vi "GetSerialNumber.vi"(8 "error in (no error)":errorcluster) -> (0 "error out":errorcluster, 2 "SerialNumber":string)   [LabVIEW 2014]
uses:
  USBAnalyzerEllisysDll.dll
panel:
  in  "stringOut":string
  in  "sizeOut 2":i32
  out "sizeOut":i32
  in  "return type":i32
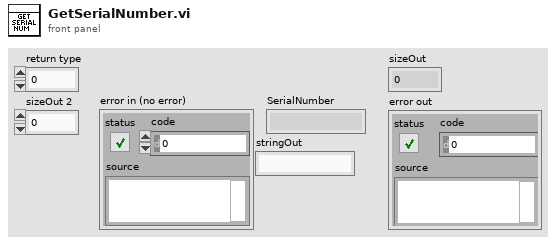
[diagram p1: front panel]
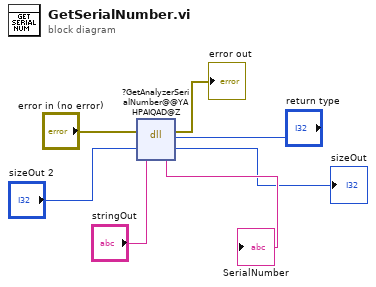
[diagram p0: block diagram]
diagram:
  n1 = dll-call lib="PTH2labs CUsersMichał\tDocumentsEllisysAnalyzerUSBAnalyzerEllisysDllDebugUSBAnalyzerEllisysDll.dll" fn="?GetAnalyzerSerialNumber@@YAHPAIQAD@Z"(error in="error in (no error)", "return type"="return type", "sizeOut"="sizeOut 2", "stringOut"="stringOut") -> (error out=→"error out":errorcluster, "sizeOut"=→"sizeOut":i32, "stringOut"=→"SerialNumber":string)  [unwired: 2 in, 1 out]
